vi "AthenaXboxUDP.vi"() -> (2 "R Thumb":i32(slide) scale=-32768.0..32768.0)   [LabVIEW 2009]
uses:
  UPD Xbox.ctl
  <vilib>/Utility/inputDevices.llb/closeJoystick.vi
  <vilib>/Utility/inputDevices.llb/joystickAcquire.vi
panel:
  in  "Millisecond Delay":u32=70
  in  "Tab Control":T1(tab)
  in  "Enable Hardware Controler":bool
  out "A":bool caption="Boolean"
  out "B":bool
  out "X":bool
  out "Y":bool
  out "RB":bool
  out "LB":bool
  out "LThumb":i32(slide) scale=-32768.0..32768.0
  out "Left Thumb button":bool
  out "Cluster":T2
  out "Left Trigger":bool
  out "Right trigger":bool
  out "Stop/Back":bool
  out "Right Thumb button":bool
  out "Direction Info":T3
  out "Z axis rotation":i32
  out "Axis Info":T4
  out "Button Info":T5
  out "Joystick Info":T6(array[cluster])
  in  "device index":i32
  out "key info":T7(array[cluster])
  out "mouse info":T8(array[cluster])
  in  "Local Port":u16=61556
  in  "Output Cluster":T9 {"Y axis\nrotation" scale=-32700.0..32700.0; "X axis\nrotation" scale=-32700.0..32700.0; "Z axis" scale=-32700.0..32700.0; "Y axis" scale=-32700.0..32700.0; "X axis" scale=-32700.0..32700.0}
  in  "Remote Port":u16=61557
  in  "Remote Host":string="localhost"
  in  "broadcast":bool
  out "type string":i16[](array[numeric])
  in  "Stop":bool
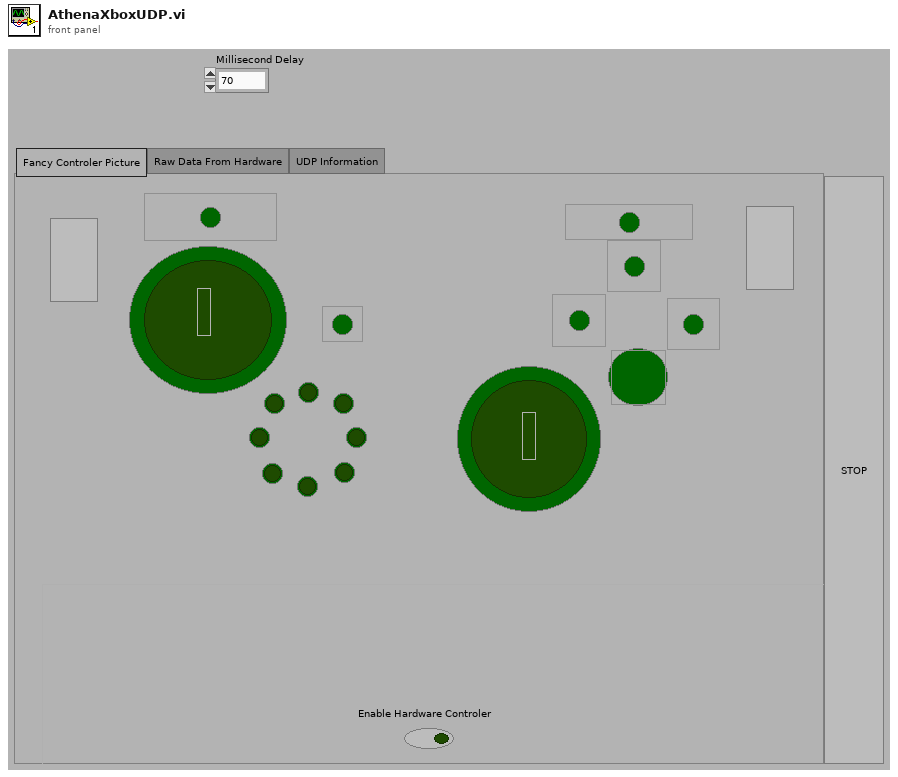
[diagram p1: front panel]
types:
  T1 = enum32{"Fancy Controler Picture", "Raw Data From Hardware", "UDP Information"}
  T2 = cluster{"Boolean 4":bool, "Boolean 6":bool, "Boolean 3":bool, "Boolean 7":bool, "Boolean 2":bool, "Boolean 9":bool, "Boolean 5":bool, "Boolean 8":bool}
  T3 = cluster{"pov 1":i32, "pov 2":i32, "pov 3":i32, "pov 4":i32}
  T4 = cluster{"X axis":i32, "Y axis":i32, "Z axis":i32, "X axis rotation":i32, "Y axis rotation":i32, "Z axis rotation":i32, "U axis":i32, "V axis":i32}
  T5 = cluster{"button 1":bool, "button 2":bool, "button 3":bool, "button 4":bool, "button 5":bool, "button 6":bool, "button 7":bool, "button 8":bool, "button 9":bool, "button 10":bool, "button 11":bool, "button 12":bool, "button 13":bool, "button 14":bool, "button 15":bool, "button 16":bool, "button 17":bool, "button 18":bool, "button 19":bool, "button 20":bool, "button 21":bool, "button 22":bool, "button 23":bool, "button 24":bool, "button 25":bool, "button 26":bool, "button 27":bool, "button 28":bool, "button 29":bool, "button 30":bool, "button 31":bool, "button 32":bool}
  T6 = cluster{"axes total":u32, "buttons total":u32, "pov total":u32, "device name":string}[]
  T7 = cluster{"buttons total":u32, "device name":string}[]
  T8 = cluster{"axes total":u32, "buttons total":u32, "device name":string}[]
  T9 = typedef "UPD Xbox.ctl" = cluster{"B":bool, "A":bool, "Y":bool, "X":bool, "X axis":i32, "Y axis":i32, "Z axis":i32, "X axis\nrotation":i32, "Y axis\nrotation":i32, "Left Bumper":bool, "Right  Bumper":bool, "Left Thumb Button":bool, "Right Thumb Button":bool, "Stop/Back":bool, "Select":bool, "Pov Angle":i32}
  T10 = cluster{"Array[0]":bool, "Array[1]":bool, "Array[2]":bool, "Array[3]":bool, "Array[4]":bool, "Array[5]":bool, "Array[6]":bool, "Array[7]":bool}
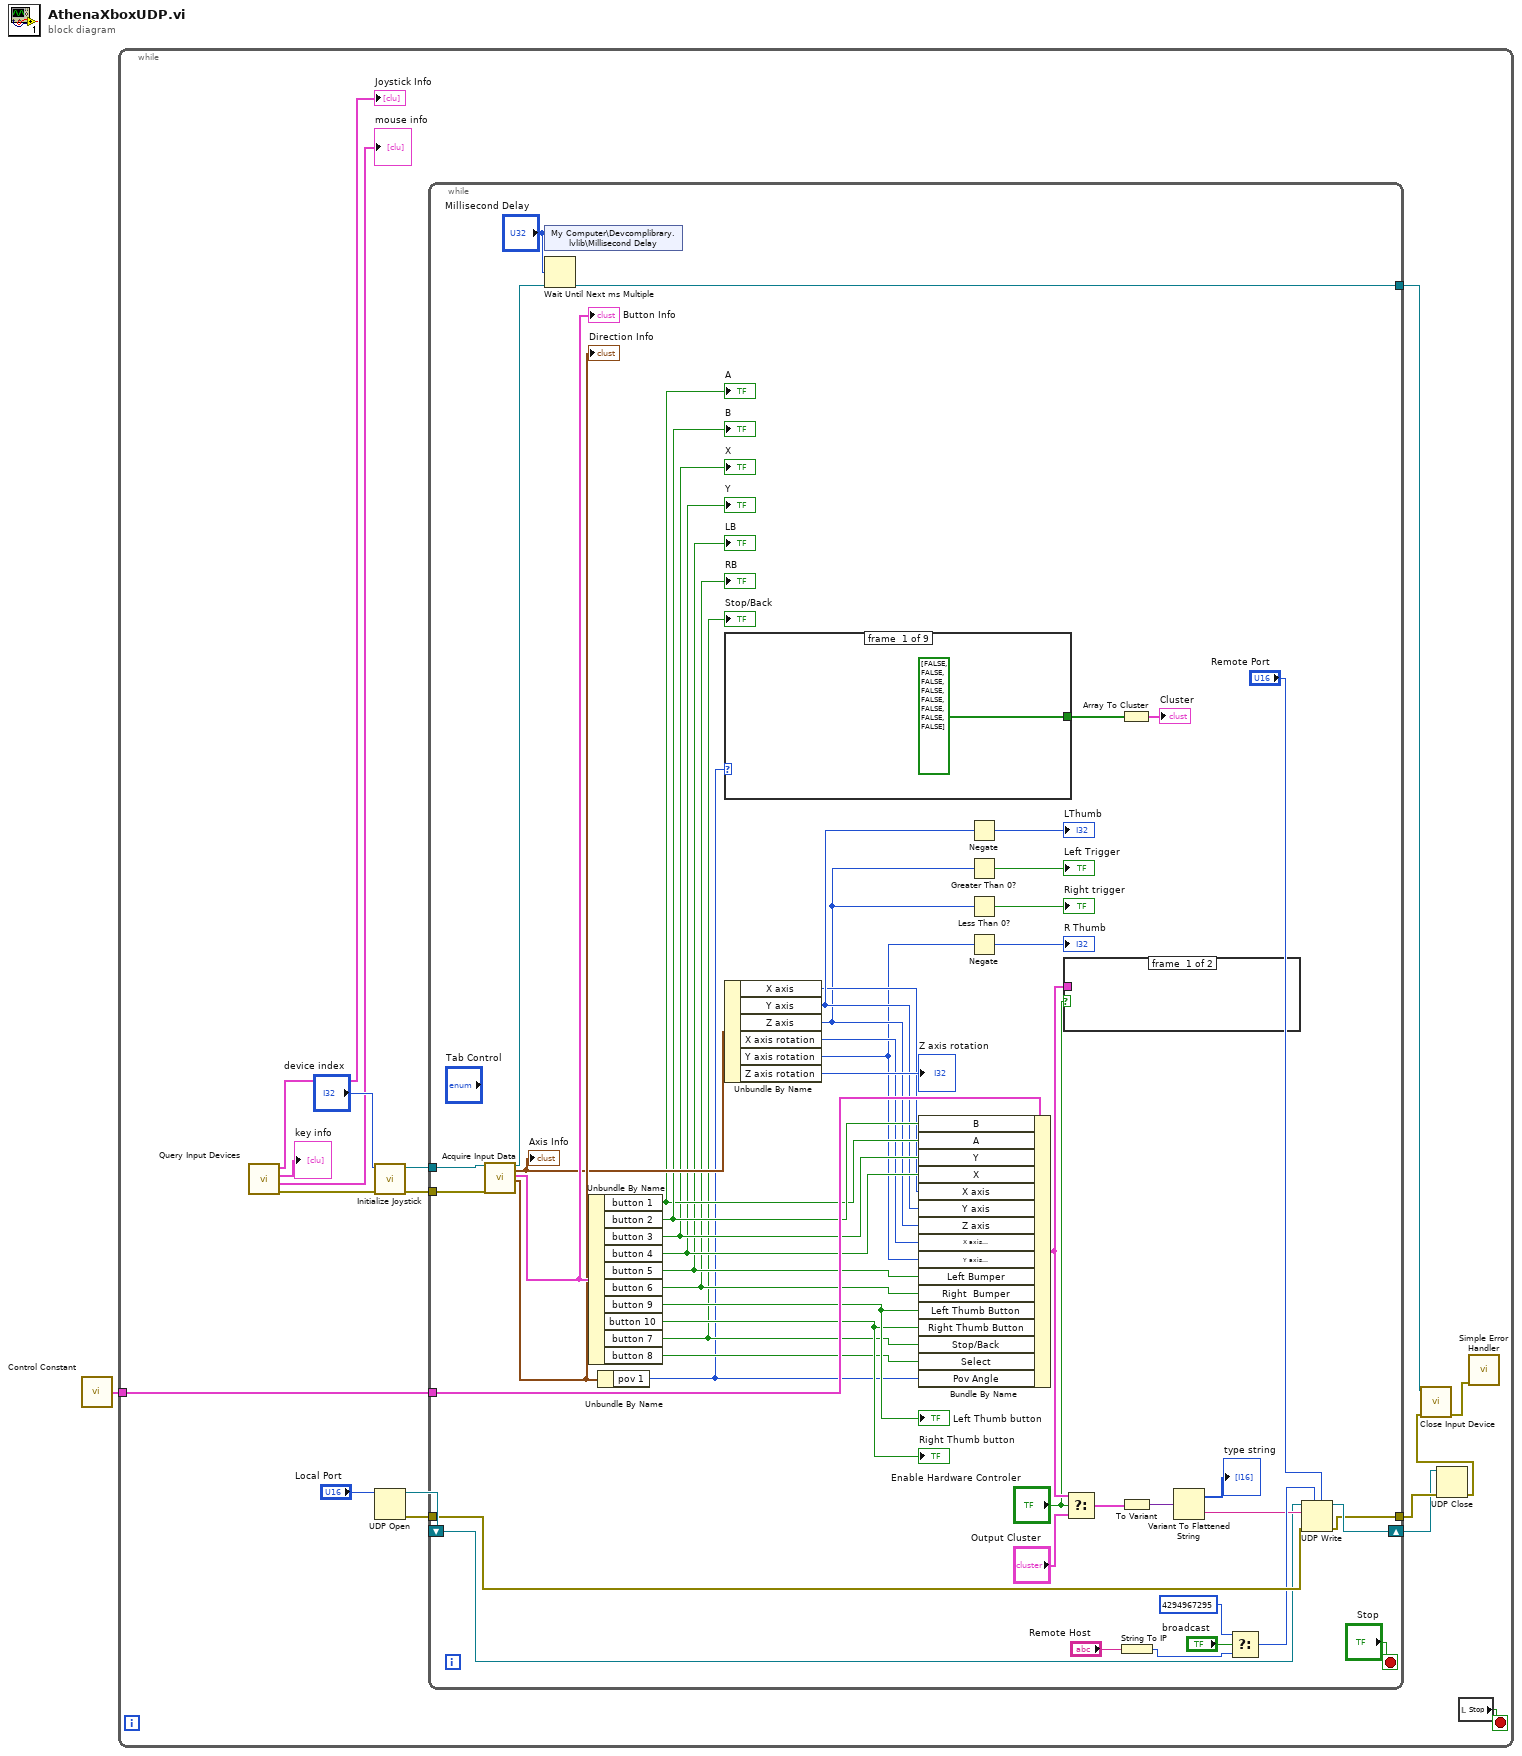
[diagram p0: block diagram]
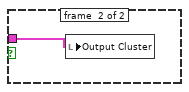
[diagram p2: hidden frame]
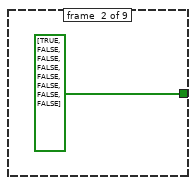
[diagram p3: hidden frame]
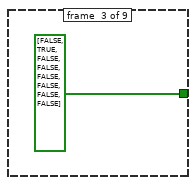
[diagram p4: hidden frame]
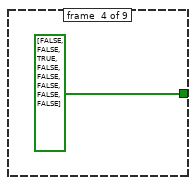
[diagram p5: hidden frame]
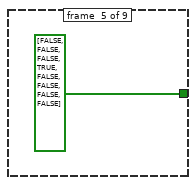
[diagram p6: hidden frame]
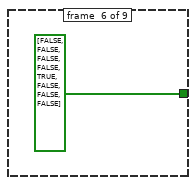
[diagram p7: hidden frame]
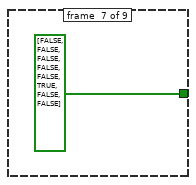
[diagram p8: hidden frame]
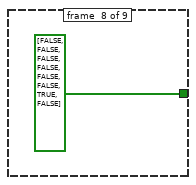
[diagram p9: hidden frame]
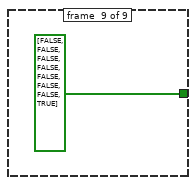
[diagram p10: hidden frame]
diagram:
  n1 = call "Control Constant.vi"() -> ("Cluster"=w1:T9)
  n2 = while {
    tunnel: w1 -> [w8]
    stop <- w11 stop-if-true
    n3 = call <vilib>:"Query Input Devices.vi"() -> ("error out"=w13:errorcluster, "mouse info"=→"mouse info":T8, "key info"=→"key info":T7, "joystick info"=→"Joystick Info":T6)  [unwired: 1 in, 7 out]
    n4 = call <vilib>:"Initialize Joystick.vi"("error in (no error)"=w13, "device index"="device index") -> ("error out"=w16:errorcluster, "device ID"=w17:refnum<k1>)  [unwired: 8 out]
    n5 = UDP Open(11:"Local Port") -> (port=w5:refnum<k16>, 0:w6:errorcluster)  [unwired: 1 in, 4 out]
    n6 = while {
      tunnel: w17 -> [w67]
      tunnel: w16 -> [w66]
      tunnel: [w65] -> w15
      tunnel: w8 -> [w53]
      tunnel: w6 -> [w29]
      shift-right: [w25] -> w3
      shift-left: w5 -> [w24]
      tunnel: [w23] -> w4
      stop <- "Stop" stop-if-true
      n7 = call-poly <vilib>:"Acquire Input Data.vi"("device ID"=w67, "error in (no error)"=w66) -> ("device ID"=w65:refnum<k1>, "axis info"=w59:T4, "button info"=w64:T5, "direction info"=w63:T3)  [unwired: 14 out]
      "Axis Info" <- w59
      "Button Info" <- w64
      "Direction Info" <- w63
      n8 = shared-variable "My Computer\\Devcomplibrary.lvlib\\Millisecond Delay"("Millisecond Delay") -> ()  [unwired: 1 in, 1 out]
      n9 = Wait Until Next ms Multiple(millisecond multiple="Millisecond Delay") -> ()  [unwired: 1 out]
      n10 = Unbundle By Name(w64) -> ("button 1"=w51:bool, "button 2"=w52:bool, "button 3"=w50:bool, "button 4"=w49:bool, "button 5"=w43:bool, "button 6"=w42:bool, "button 9"=w41:bool, "button 10"=w40:bool, "button 7"=w39:bool, "button 8"=w38:bool)
      "A" <- w51
      "B" <- w52
      "Y" <- w49
      "X" <- w50
      "RB" <- w42
      "LB" <- w43
      "Left Thumb button" <- w41
      "Right Thumb button" <- w40
      "Stop/Back" <- w39
      n11 = Unbundle By Name(w63) -> ("pov 1"=w37:i32)
      n12 = case shown="0" w37 {
        tunnel: [bool[] [FALSE, FALSE, FALSE, FALSE, FALSE, FALSE, FALSE, FALSE] ("Array") bool[] [TRUE, FALSE, FALSE, FALSE, FALSE, FALSE, FALSE, FALSE] ("Array") bool[] [FALSE, TRUE, FALSE, FALSE, FALSE, FALSE, FALSE, FALSE] ("Array") bool[] [FALSE, FALSE, TRUE, FALSE, FALSE, FALSE, FALSE, FALSE] ("Array") bool[] [FALSE, FALSE, FALSE, TRUE, FALSE, FALSE, FALSE, FALSE] ("Array") bool[] [FALSE, FALSE, FALSE, FALSE, TRUE, FALSE, FALSE, FALSE] ("Array") bool[] [FALSE, FALSE, FALSE, FALSE, FALSE, TRUE, FALSE, FALSE] ("Array") bool[] [FALSE, FALSE, FALSE, FALSE, FALSE, FALSE, TRUE, FALSE] ("Array") bool[] [FALSE, FALSE, FALSE, FALSE, FALSE, FALSE, FALSE, TRUE] ("Array")] -> w55
        frame #0 {
        }
        frame #1 {
        }
        frame #2 {
        }
        frame #3 {
        }
        frame #4 {
        }
        frame #5 {
        }
        frame #6 {
        }
        frame #7 {
        }
        frame #8 {
        }
      }
      n13 = Unbundle By Name(w59) -> ("X axis"=w47:i32, "Y axis"=w48:i32, "Z axis"=w46:i32, "X axis rotation"=w45:i32, "Y axis rotation"=w44:i32, "Z axis rotation"=→"Z axis rotation":i32)
      n14 = Bundle By Name(cluster=w53, "B"=w52, "A"=w51, "Y"=w50, "X"=w49, "X axis"=w47, "Y axis"=w48, "Z axis"=w46, "X axis\nrotation"=w45, "Y axis\nrotation"=w44, "Left Bumper"=w43, "Right  Bumper"=w42, "Left Thumb Button"=w41, "Right Thumb Button"=w40, "Stop/Back"=w39, "Select"=w38, "Pov Angle"=w37) -> (w20:T9)
      n15 = Negate(x=w48) -> (-x=→"LThumb":i32)
      n16 = Greater Than 0?(x=w46) -> (x > 0?=→"Left Trigger":bool)
      n17 = Less Than 0?(x=w46) -> (x < 0?=→"Right trigger":bool)
      n18 = Negate(x=w44) -> (-x=→"R Thumb":i32)
      n19 = case shown="True" "Enable Hardware Controler" {
        tunnel: w20 -> [_ w68]
        frame #0 {
        }
        frame #1 {
          n20 = local write "Output Cluster"(w68) -> ()
        }
      }
      n21 = Select(t=w20, s="Enable Hardware Controler", f="Output Cluster") -> (s? t:f=w22:T9)
      n22 = Array To Cluster(array=w55) -> (cluster=→"Cluster":T10)
      n23 = To Variant(anything=w22) -> (Variant=w36:variant)
      n24 = String To IP(1:"Remote Host") -> (0:w33:u32)
      n25 = Variant To Flattened String(Variant=w36) -> (data string=w26:string, 1:→"type string":i16[])
      n26 = Select(t=u32 4294967295, s="broadcast", f=w33) -> (s? t:f=w28:u32)
      n27 = UDP Write(address=w28, port or service name="Remote Port", connection ID=w24, data in=w26, 8:w29) -> (error out=w23:errorcluster, 3:w25:refnum<k16>)  [unwired: 1 out]
    }
    n28 = UDP Close(connection ID=w3, 8:w4) -> (error out=w2:errorcluster)  [unwired: 1 out]
    n29 = call-poly <vilib>:"Close Input Device.vi"("error in (no error)"=w2, "device ID"=w15) -> ("error out"=w12:errorcluster)  [unwired: 8 out]
    n30 = local read "Stop"() -> (w11:bool)
    n31 = call <vilib>:"Simple Error Handler.vi"("error in (no error)"=w12) -> ()  [unwired: 1 in, 8 out]
  }
